vi "Task Cluster.vi"(8 "error in (no error)":errorcluster, 11 "Task Config in":refnum<class "Task Config.lvclass">) -> (0 "error out":errorcluster, 2 "Cluster":refnum<class "Cluster Config.lvclass">, 3 "Task Config out":refnum<class "Task Config.lvclass">)   [LabVIEW 2020, in "VolatusConfig.lvlib"]
uses:
  VolatusConfig.lvlib
  Task/Task Config.lvclass
  C:/dev/lv20CE/relink/lv-volatus/VolatusConfig/VolatusConfigElement/VolatusConfigElement.lvclass
  Cluster/Cluster Config.lvclass
  Meta Type.ctl
  VolatusConfigElement/VolatusConfigElement.lvclass/VolatusConfigElement.ctl
  VolatusConfigElement/Element.vi
  lv-cdm/CDM-Config/Config Lookup/Match Meta.vi
  lv-cdm/CDM-Config/Config Element/Owner.vi
  lv-cdm/CDM-Config/Config Filter/Config Lookup.lvclass
  VolatusConfigElement/VolatusConfigElement.lvclass
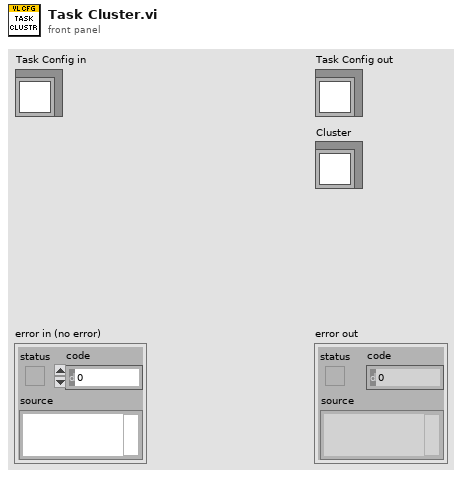
[diagram p1: front panel]
types:
  T1 = typedef "VolatusConfig.lvlib/Meta Type.ctl" = enum16{"UNKNOWN", "VL_System", "VL_Cluster", "VL_Node", "VL_Task", "VL_Group", "VL_Channel", "VL_Task_List", "VL_Scaling", "VL_Sensor", "VL_Sensor_List", "VL_Scale"}
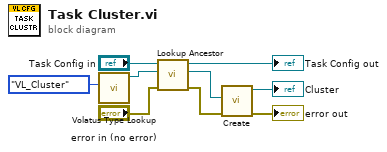
[diagram p0: block diagram]
diagram:
  n1 = call "Volatus Type Lookup.vi"("Meta Type"=Meta_Type."VL_Cluster") -> ("Config Lookup out"=w9:refnum<class "Config Lookup.lvclass">)  [unwired: 9 in, 1 out]
  n2 = call "Lookup Ancestor.vi"("error in (no error)"="error in (no error)", "Lookup"=w9, "VolatusConfigElement in"="Task Config in") -> ("error out"=w3:errorcluster, "Ancestor"=w7:refnum<class "Config Element.lvclass">, "VolatusConfigElement out"=→"Task Config out":refnum<class "Task Config.lvclass">)  [unwired: 6 in]
  n3 = call "Create.vi"("error in (no error)"=w3, "Element"=w7) -> ("error out"=→"error out":errorcluster, "Cluster out"=→"Cluster":refnum<class "Cluster Config.lvclass">)  [unwired: 8 in]
